vi "Update Line Inversion.vi"(8 "error in (no error)":errorcluster, 9 "Output Line":i32, 10 "Invert Line":bool, 11 "Master Device in":refnum<class "Master Device.lvclass">) -> (0 "error out":errorcluster, 3 "Master Device out":refnum<class "Master Device.lvclass">)   [LabVIEW 2013, in "Master Device.lvclass"]
uses:
  Master Device.lvclass
  Master Device.lvclass/Master Device.ctl
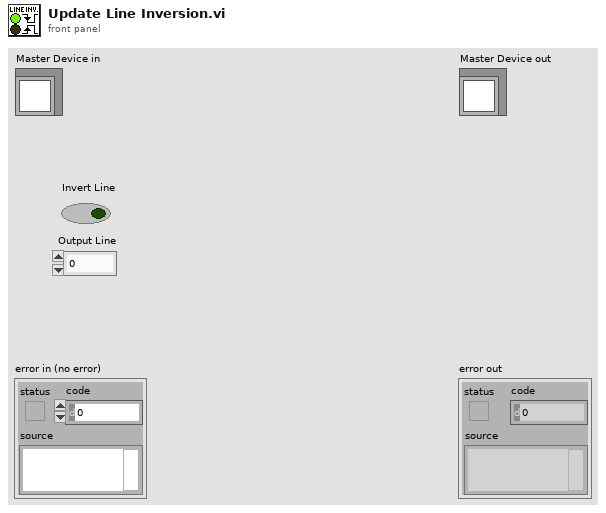
[diagram p1: front panel]
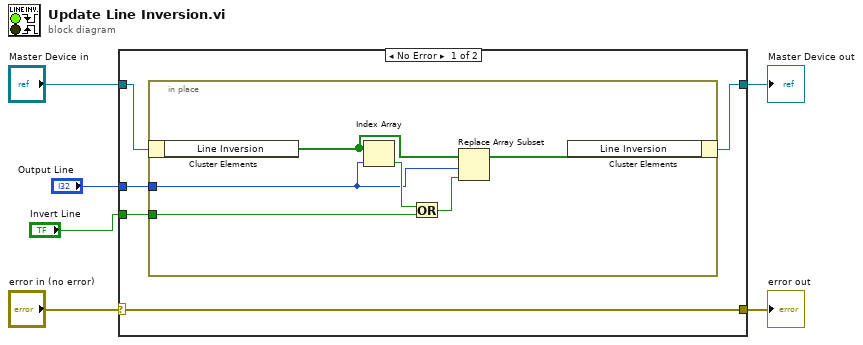
[diagram p0: block diagram]
diagram:
  n1 = case shown="No Error" "error in (no error)" {
    selector: "error in (no error)" -> [w11 w18]
    tunnel: [w11 w18] -> w5
    tunnel: [w9 w19] -> w3
    tunnel: "Master Device in" -> [w10 w19]
    tunnel: "Output Line" -> [w8 _]
    tunnel: "Invert Line" -> [w7 _]
    frame No Error {
      n2 = in-place {
        in-place-border: w7 -> [w16]
        in-place-border: w8 -> [w12]
        n3 = in-place-cluster #1(w10) -> ("Line Inversion"=w15:bool[])
        n4 = Index Array(array=w15, index=w12) -> (element=w17:bool)
        n5 = Or(x=w17, y=w16) -> (x .or. y?=w13:bool)
        n6 = Replace Array Subset(array=w15, new element=w13, index=w12) -> (w14:bool[])
        n7 = in-place-cluster #1("Line Inversion"=w14) -> (w9:refnum<class "Master Device.lvclass">)
      }
    }
    frame Error {
    }
  }
  "error out" <- w5
  "Master Device out" <- w3
